vi "Teleop.vi"(10 "Match Info":T1={"Autonomous Elapsed Seconds"=0.0, "TeleOp Elapsed Seconds"=0.0, "Disabled Elapsed Seconds"=0.0, "Visited Autonomous"=FALSE, "Visited TeleOp"=FALSE, "Visited Disabled"=FALSE, "Autonomous Settings"={"Autonomous Style"=enum."Independent", "VI Refnum"=refnum}}, 11 "Call Context":T2) -> ()   [LabVIEW 2016]
doc: "This VI is called for each TeleOp packet received from the DS where the robot is not disabled. It is often used to read from the joysticks and update I/O or to update setpoints for timed control loops. It should complete and return within 20 milliseconds or it may miss DS packets."
uses:
  <vilib>/Rock Robotics/WPI/DriverStation/WPI_DriverStationDerivedRobotMode.ctl
  <vilib>/Rock Robotics/WPI/DriverStation/WPI_DriverStationMatch Info.ctl
  <vilib>/Rock Robotics/WPI/Relay/WPI_RelayValue.ctl
  <vilib>/Rock Robotics/WPI/Utilities/WPI_GetSetVariantRefNum.vi
  <vilib>/Rock Robotics/Network Tables/NT Write Boolean Array.vi
  <vilib>/Rock Robotics/Network Tables/NT Write Numeric Array.vi
  <vilib>/Rock Robotics/Network Tables/NT Read Boolean.vi
  <vilib>/Rock Robotics/Network Tables/NT Read Number.vi
  Robot Global Data.vi
panel:
  out "size y (1-200)":dbl
  out "center y (0-119)":dbl
  out "x+1":i32
  out "Sample Slider 0":dbl(slide) scale=0.0..5.0
  out "Sample Boolean 1":bool
  out "Sample Boolean 0":bool
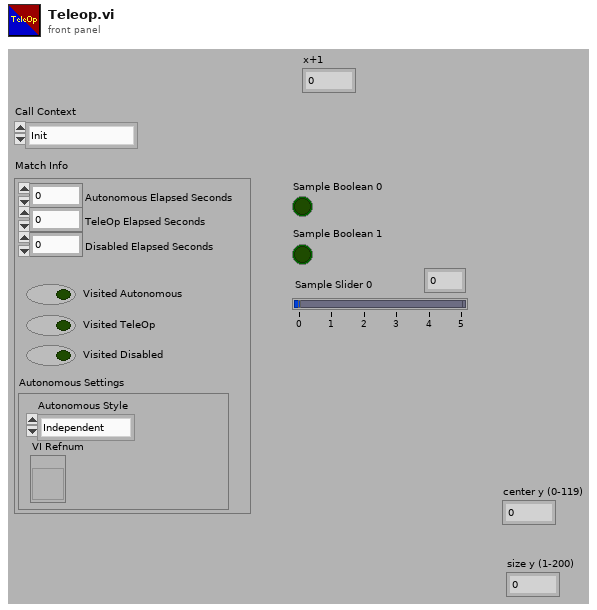
[diagram p1: front panel]
types:
  T1 = typedef "WPI_DriverStationMatch Info.ctl" = cluster{"Autonomous Elapsed Seconds":dbl, "TeleOp Elapsed Seconds":dbl, "Disabled Elapsed Seconds":dbl, "Visited Autonomous":bool, "Visited TeleOp":bool, "Visited Disabled":bool, "Autonomous Settings":cluster{"Autonomous Style":enum16{"Iterative", "Independent"}, "VI Refnum":refnum<vi>}}
  T2 = typedef "WPI_DriverStationDerivedRobotMode.ctl" = enum16{"Init", "Execute", "Stop"}
  T3 = typedef "WPI_RelayValue.ctl" = enum16{"Off", "On", "Forward", "Reverse"}
  T4 = typedef "WPI_JoystickDevRef.ctl" = cluster{"Device":T5}
  T5 = typedef "WPI_JoystickDeviceEnum.ctl" = enum16{"USB 0", "USB 1", "USB 2", "USB 3", "USB 4", "USB 5"}
  T6 = cluster{"Axes[0]":dbl, "Axes[1]":dbl, "Axes[2]":dbl, "Axes[3]":dbl, "Axes[4]":dbl, "Axes[5]":dbl, "Axes[6]":dbl, "Axes[7]":dbl, "Axes[8]":dbl}
  T7 = cluster{"Buttons[0]":bool, "Buttons[1]":bool, "Buttons[2]":bool, "Buttons[3]":bool, "Buttons[4]":bool, "Buttons[5]":bool, "Buttons[6]":bool, "Buttons[7]":bool, "Buttons[8]":bool}
  T8 = typedef "WPI_MotorControlDeviceRef.ctl" = cluster{"DeviceStatus":errorcluster, "Type":T9, "PWM":cluster{"PWM Channel":T10, "DeadBand":T11}, "CAN":cluster{"Device Number":u8, "SetOutput VI Ref":variant, "GetOutput VI Ref":variant, "Enable VI Ref":variant, "Disable VI Ref":variant, "Data":variant}, "Invert":bool}
  T9 = typedef "WPI_MotorControlType.ctl" = enum16{"PWM", "CAN"}
  T10 = typedef "FPGA_DIOPWMChannel.ctl" = enum8{"PWM 0", "PWM 1", "PWM 2", "PWM 3", "PWM 4", "PWM 5", "PWM 6", "PWM 7", "PWM 8", "PWM 9", "PWM MXP 0", "PWM MXP 1", "PWM MXP 2", "PWM MXP 3", "PWM MXP 4", "PWM MXP 5", "PWM MXP 6", "PWM MXP 7", "PWM MXP 8", "PWM MXP 9", "Invalid"}
  T11 = typedef "WPI_PWMDeadband.ctl" = cluster{"Name":string, "maxPositivePwm":i32, "minPositivePwm":i32, "centerPwm":i32, "maxNegativePwm":i32, "minNegativePwm":i32, "angularRange":u16}
  T12 = typedef "WPI_RelayDevRef.ctl" = cluster{"DevStatus":errorcluster, "Relay Channel":T13, "Relay Direction":T14}
  T13 = typedef "FPGA_DIORelayChannel.ctl" = enum8{"Relay 0", "Relay 1", "Relay 2", "Relay 3", "Invalid"}
  T14 = typedef "WPI_RelayDirection.ctl" = enum16{"Both directions", "Forward only", "Reverse only"}
  T15 = typedef "WPI_RobotDriveDevRef.ctl" = cluster{"DevStatus":errorcluster, "Motors[]":T8[], "Square Inputs":bool, "Max Output":dbl}
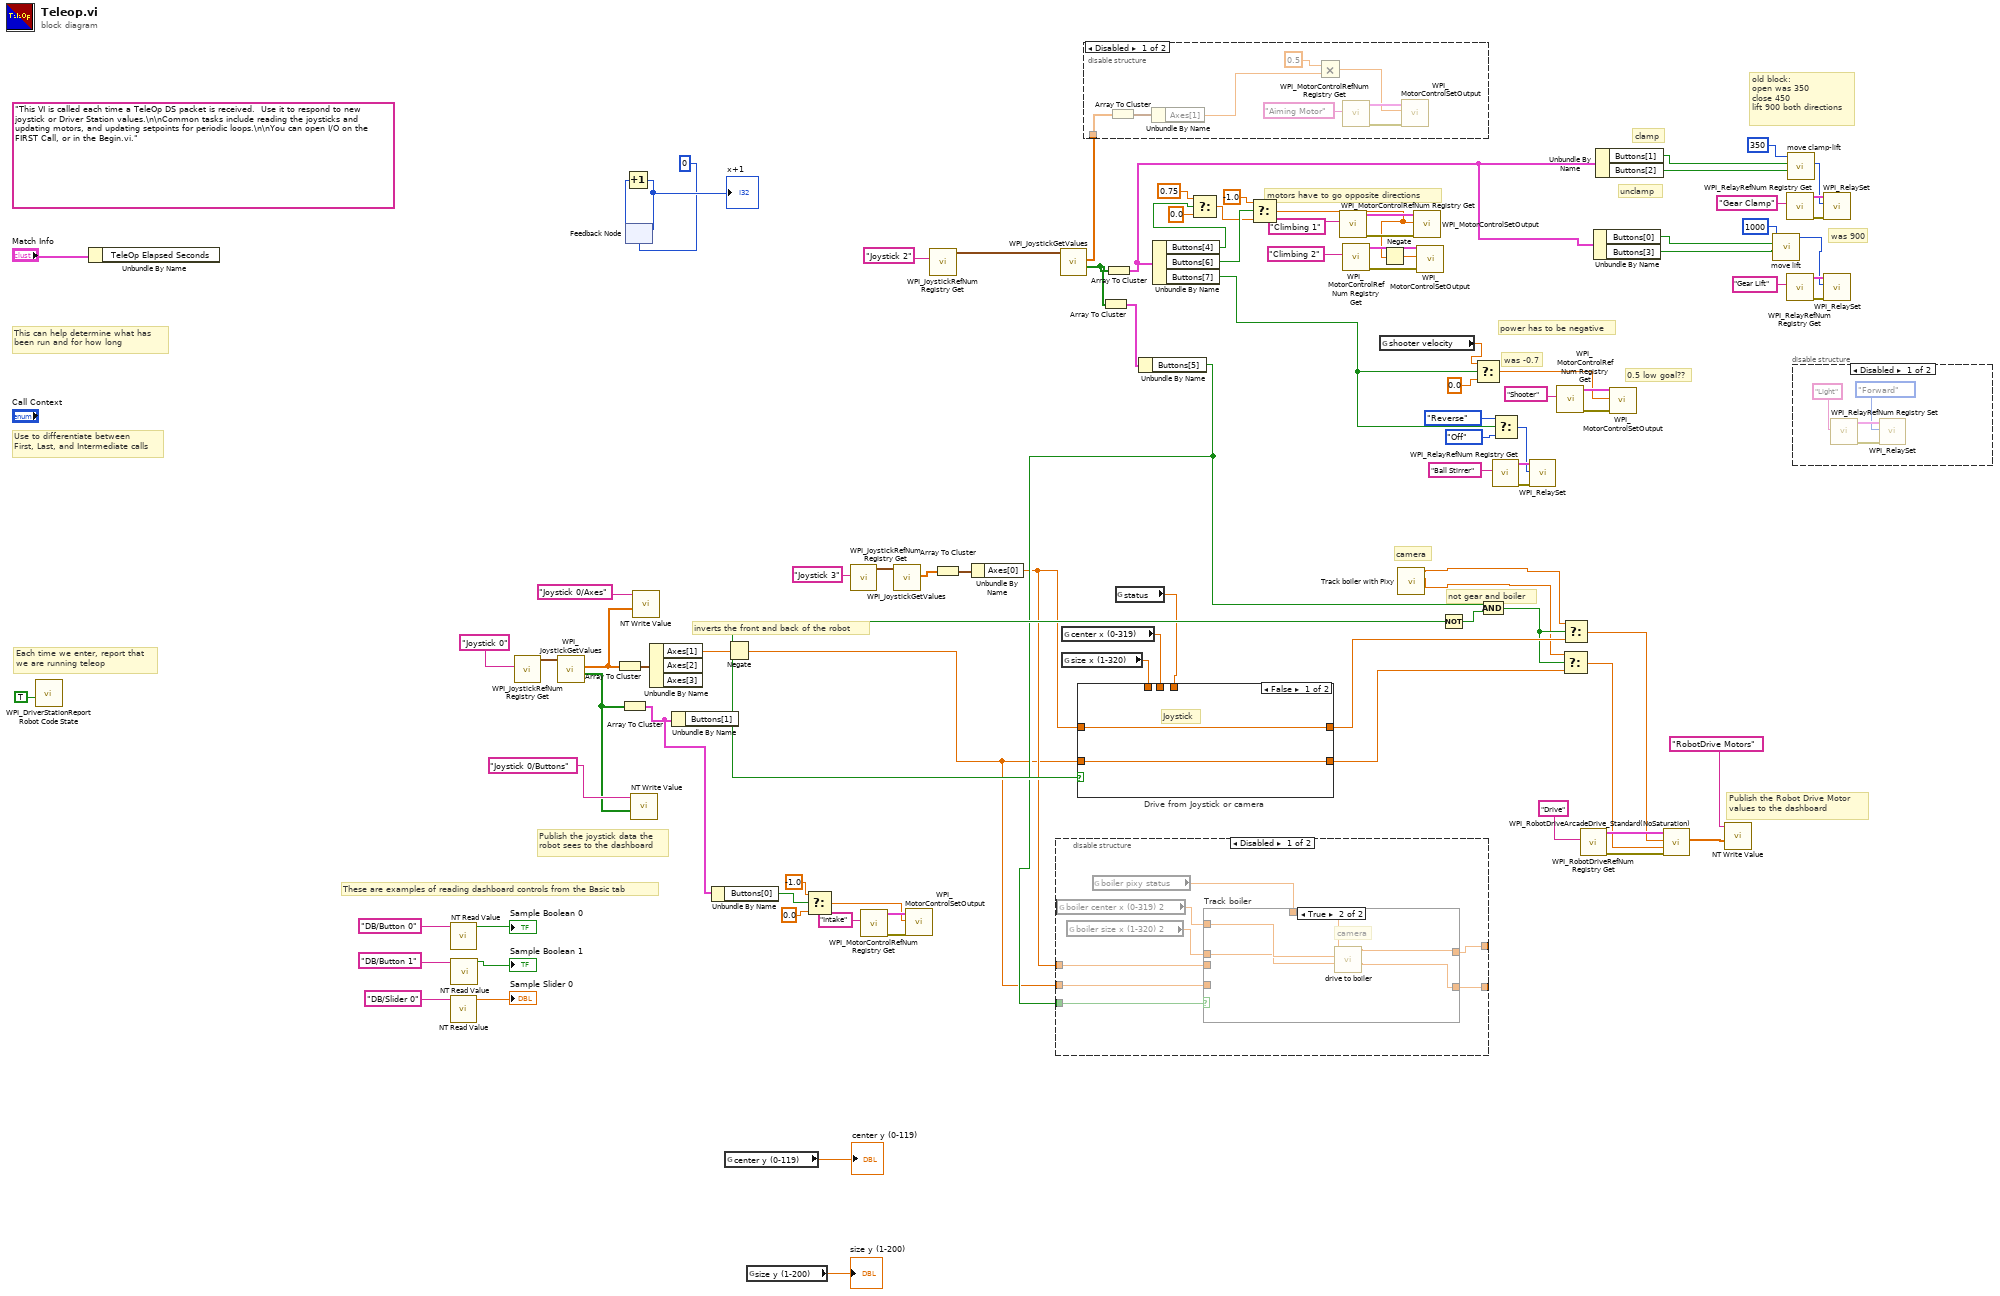
[diagram p0: block diagram]
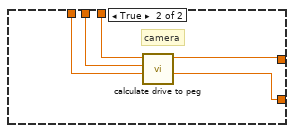
[diagram p6: hidden frame]
diagram:
  (unwired) "This VI is called each time a TeleOp DS packet is received.  Use it to respond to new joystick or Driver Station values.\n\nCommon tasks include reading the joysticks and updating motors, and updating setpoints for periodic loops.\n\nYou can open I/O on the FIRST Call, or in the Begin.vi."
  # "camera"
  # "not gear and boiler"
  # "was 900"
  # "old block:\nopen was 350\nclose 450\nlift 900 both directions"
  # "inverts the front and back of the robot"
  # "unclamp"
  # "clamp"
  # "was -0.7"
  # "0.5 low goal??"
  # "power has to be negative"
  # "motors have to go opposite directions"
  # "These are examples of reading dashboard controls from the Basic tab"
  # "Publish the Robot Drive Motor\nvalues to the dashboard"
  # "Publish the joystick data the\nrobot sees to the dashboard"
  # "Each time we enter, report that\nwe are running teleop"
  # "Use to differentiate between\nFirst, Last, and Intermediate calls"
  # "This can help determine what has\nbeen run and for how long"
  n1 = call <vilib>:"WPI_DriverStationReport Robot Code State.vi"("TeleOp"=TRUE ("Autonomous")) -> ()  [unwired: 10 in, 1 out]
  n2 = Unbundle By Name("Match Info") -> ()  [unwired: 1 out]
  n3 = call-poly <vilib>:"NT Read Value.vi"("Name"="DB/Button 0" ("refnum name")) -> ("Boolean"=→"Sample Boolean 0":bool)  [unwired: 9 in, 1 out]
  n4 = call-poly <vilib>:"NT Read Value.vi"("Name"="DB/Slider 0" ("refnum name")) -> ("Numeric"=→"Sample Slider 0":dbl)  [unwired: 9 in, 1 out]
  n5 = call-poly <vilib>:"NT Read Value.vi"("Name"="DB/Button 1" ("refnum name")) -> ("Boolean"=→"Sample Boolean 1":bool)  [unwired: 9 in, 1 out]
  n6 = call <vilib>:"WPI_JoystickRefNum Registry Get.vi"("refnum name"="Joystick 0") -> ("JoystickDevRef"=w96:T4)  [unwired: 1 in, 9 out]
  n7 = call <vilib>:"WPI_JoystickGetValues.vi"("JoystickDevRef"=w96) -> ("Buttons"=w84:bool[], "Axes"=w85:dbl[])  [unwired: 6 in, 3 out]
  n8 = Array To Cluster(array=w85) -> (cluster=w86:T6)
  n9 = Array To Cluster(array=w84) -> (cluster=w35:T7)
  n10 = feedback #1(0) -> (w75:i32)
  n11 = Increment(x=w75) -> (x+1=w76:i32)
  "x+1" <- w76
  n12 = feedback-in #1(w76) -> ()
  n13 = call-poly <vilib>:"NT Write Value.vi"("Boolean Array"=w84, "Name"="Joystick 0/Buttons") -> ()  [unwired: 9 in, 1 out]
  n14 = call-poly <vilib>:"NT Write Value.vi"("Numeric Array"=w85, "Name"="Joystick 0/Axes") -> ()  [unwired: 9 in, 1 out]
  n15 = Unbundle By Name(w86) -> ("Axes[1]"=w73:dbl)  [unwired: 2 out]
  n16 = Unbundle By Name(w35) -> ("Buttons[1]"=w20:bool)
  n17 = Unbundle By Name(w35) -> ("Buttons[0]"=w33:bool)
  n18 = global read "Robot Global Data.vi" "center y (0-119)"() -> (→"center y (0-119)":dbl)
  n19 = Negate(x=w73) -> (-x=w13:dbl)
  n20 = global read "Robot Global Data.vi" "size y (1-200)"() -> (→"size y (1-200)":dbl)
  n21 = Select(t=-1.0, s=w33, f=0.0) -> (s? t:f=w78:dbl)
  n22 = call <vilib>:"WPI_JoystickRefNum Registry Get.vi"("refnum name"="Joystick 3") -> ("JoystickDevRef"=w45:T4)  [unwired: 1 in, 9 out]
  n23 = call <vilib>:"WPI_MotorControlRefNum Registry Get.vi"("refnum name"="Intake") -> ("error out"=w81:errorcluster, "MotorControlDevRef"=w80:T8)  [unwired: 9 in]
  n24 = call <vilib>:"WPI_JoystickGetValues.vi"("JoystickDevRef"=w45) -> ("Axes"=w44:dbl[])  [unwired: 6 in, 4 out]
  n25 = call <vilib>:"WPI_MotorControlSetOutput.vi"("error in (no error)"=w81, "Output"=w78, "MotorControlDevRef"=w80) -> ()  [unwired: 6 in, 3 out]
  n26 = call <vilib>:"WPI_JoystickRefNum Registry Get.vi"("refnum name"="Joystick 2") -> ("JoystickDevRef"=w68:T4)  [unwired: 1 in, 9 out]
  n27 = Array To Cluster(array=w44) -> (cluster=w43:T6)
  n28 = Unbundle By Name(w43) -> ("Axes[0]"=w14:dbl)
  n29 = call <vilib>:"WPI_JoystickGetValues.vi"("JoystickDevRef"=w68) -> ("Buttons"=w19:bool[], "Axes"=w60:dbl[])  [unwired: 6 in, 3 out]
  n30 = global read "Robot Global Data.vi" "center x (0-319)"() -> (w11:dbl)
  n31 = global read "Robot Global Data.vi" "size x (1-320)"() -> (w10:dbl)
  n32 = disable-structure shown="Disabled" {
    disable-tunnel: w60 -> [w108 _]
    frame Disabled {
      n33 = Array To Cluster(array=w108) -> (cluster=w107:T6)
      n34 = Unbundle By Name(w107) -> ("Axes[1]"=w101:dbl)
      n35 = Multiply(x=0.5 ("y"), y=w101) -> (x*y=w103:dbl)
      n36 = call <vilib>:"WPI_MotorControlRefNum Registry Get.vi"("refnum name"="Aiming Motor") -> ("error out"=w104:errorcluster, "MotorControlDevRef"=w105:T8)  [unwired: 9 in]
      n37 = call <vilib>:"WPI_MotorControlSetOutput.vi"("error in (no error)"=w104, "Output"=w103, "MotorControlDevRef"=w105) -> ()  [unwired: 6 in, 3 out]
    }
    frame Enabled {
    }
  }
  n38 = Array To Cluster(array=w19) -> (cluster=w16:T7)
  n39 = Array To Cluster(array=w19) -> (cluster=w18:T7)
  n40 = global read "Robot Global Data.vi" "status"() -> (w12:dbl)
  n41 = case "Drive from Joystick or camera" shown="False" w20 {
    tunnel: w14 -> [w110 _]
    tunnel: [w110 w115] -> w9
    tunnel: w13 -> [w109 _]
    tunnel: [w109 w114] -> w8
    tunnel: w12 -> [_ w113]
    tunnel: w11 -> [_ w112]
    tunnel: w10 -> [_ w111]
    frame False {
      # "Joystick"
    }
    frame True {
      # "camera"
      n42 = call "calculate drive to peg.vi"("status"=w113, "center x (0-319)"=w112, "size x (1-320)"=w111) -> ("x"=w115:dbl, "y"=w114:dbl)  [unwired: 6 in]
    }
  }
  n43 = Unbundle By Name(w16) -> ("Buttons[5]"=w15:bool)
  n44 = disable-structure shown="Disabled" {
    disable-tunnel: w15 -> [w120 _]
    disable-tunnel: [w119 _] -> _
    disable-tunnel: [w118 _] -> _
    disable-tunnel: w14 -> [w117 _]
    disable-tunnel: w13 -> [w116 _]
    frame Disabled {
      n45 = global read "Robot Global Data.vi" "boiler center x (0-319) 2"() -> (w122:dbl)
      n46 = global read "Robot Global Data.vi" "boiler size x (1-320) 2"() -> (w121:dbl)
      n47 = global read "Robot Global Data.vi" "boiler pixy status"() -> (w123:dbl)
      n48 = case "Track boiler" shown="True" w120 {
        tunnel: [w125 w130] -> w119
        tunnel: [w124 w129] -> w118
        tunnel: w123 -> [_ w128]
        tunnel: w122 -> [_ w127]
        tunnel: w121 -> [_ w126]
        tunnel: w117 -> [w125 _]
        tunnel: w116 -> [w124 _]
        frame False {
          # "Joystick"
        }
        frame True {
          # "camera"
          n49 = call "drive to boiler.vi"(9:w126, 10:w127, 11:w128) -> ("y output"=w129:dbl, "x output"=w130:dbl)  [unwired: 7 in]
        }
      }
    }
    frame Enabled {
    }
  }
  n50 = Unbundle By Name(w18) -> ("Buttons[4]"=w27:bool, "Buttons[6]"=w41:bool, "Buttons[7]"=w17:bool)
  n51 = Select(t=0.75, s=w27, f=0.0) -> (s? t:f=w25:dbl)
  n52 = Select(t=-1.0, s=w41, f=w25) -> (s? t:f=w36:dbl)
  n53 = call <vilib>:"WPI_MotorControlRefNum Registry Get.vi"("refnum name"="Climbing 1") -> ("error out"=w66:errorcluster, "MotorControlDevRef"=w65:T8)  [unwired: 9 in]
  n54 = call <vilib>:"WPI_MotorControlRefNum Registry Get.vi"("refnum name"="Climbing 2") -> ("error out"=w63:errorcluster, "MotorControlDevRef"=w64:T8)  [unwired: 9 in]
  n55 = global read "Robot Global Data.vi" "shooter velocity"() -> (w1:dbl)
  n56 = Negate(x=w36) -> (-x=w37:dbl)
  n57 = call "Track boiler with Pixy.vi"() -> ("y output"=w4:dbl, "x output"=w5:dbl)  [unwired: 7 in, 2 out]
  n58 = call <vilib>:"WPI_MotorControlSetOutput.vi"("error in (no error)"=w66, "Output"=w36, "MotorControlDevRef"=w65) -> ()  [unwired: 6 in, 3 out]
  n59 = call <vilib>:"WPI_MotorControlSetOutput.vi"("error in (no error)"=w63, "Output"=w37, "MotorControlDevRef"=w64) -> ()  [unwired: 6 in, 3 out]
  n60 = Not(x=w20) -> (.not. x?=w6:bool)
  n61 = Select(t=w1, s=w17, f=0.0) -> (s? t:f=w56:dbl)
  n62 = And(x=w15, y=w6) -> (x .and. y?=w7:bool)
  n63 = call <vilib>:"WPI_RelayRefNum Registry Get.vi"("refnum name"="Ball Stirrer") -> ("error out"=w54:errorcluster, "RelayDevRef"=w53:T12)  [unwired: 9 in]
  n64 = Select(t=WPI_RelayValue."Reverse" ("RelayValue"), s=w17, f=WPI_RelayValue."Off" ("RelayValue")) -> (s? t:f=w52:T3)
  n65 = call <vilib>:"WPI_RelaySet.vi"("error in (no error)"=w54, "RelayValue"=w52, "RelayDevRef"=w53) -> ()  [unwired: 7 in, 2 out]
  n66 = call <vilib>:"WPI_MotorControlRefNum Registry Get.vi"("refnum name"="Shooter") -> ("error out"=w59:errorcluster, "MotorControlDevRef"=w58:T8)  [unwired: 9 in]
  n67 = Select(t=w4, s=w7, f=w8) -> (s? t:f=w2:dbl)
  n68 = Select(t=w5, s=w7, f=w9) -> (s? t:f=w3:dbl)
  n69 = call <vilib>:"WPI_RobotDriveRefNum Registry Get.vi"("refnum name"="Drive") -> ("error out"=w34:errorcluster, "RobotDriveDevRef"=w98:T15)  [unwired: 1 in, 8 out]
  n70 = Unbundle By Name(w18) -> ("Buttons[0]"=w23:bool, "Buttons[3]"=w22:bool)
  n71 = Unbundle By Name(w18) -> ("Buttons[1]"=w31:bool, "Buttons[2]"=w30:bool)
  n72 = call <vilib>:"WPI_MotorControlSetOutput.vi"("error in (no error)"=w59, "Output"=w56, "MotorControlDevRef"=w58) -> ()  [unwired: 6 in, 3 out]
  n73 = call <vilib>:"WPI_RobotDriveArcadeDrive_Standard(NoSaturation).vi"("error in (no error)"=w34, "Y axis value"=w2, "X axis value"=w3, "RobotDriveDevRef"=w98) -> ("Motor Values"=w70:dbl[])  [unwired: 7 out]
  n74 = call-poly <vilib>:"NT Write Value.vi"("Numeric Array"=w70, "Name"="RobotDrive Motors") -> ()  [unwired: 9 in, 1 out]
  n75 = call "move lift.vi"("button 3"=w22, "button 0"=w23, "time"=u32 1000 ("forward time")) -> ("output"=w24:T3)  [unwired: 8 in]
  n76 = call <vilib>:"WPI_RelayRefNum Registry Get.vi"("refnum name"="Gear Clamp") -> ("error out"=w48:errorcluster, "RelayDevRef"=w47:T12)  [unwired: 9 in]
  n77 = call <vilib>:"WPI_RelayRefNum Registry Get.vi"("refnum name"="Gear Lift") -> ("error out"=w38:errorcluster, "RelayDevRef"=w39:T12)  [unwired: 9 in]
  n78 = call "move clamp-lift.vi"("button 2"=w30, "button 1"=w31, "time"=u32 350 ("forward time")) -> ("output"=w29:T3)  [unwired: 8 in]
  n79 = disable-structure shown="Disabled" {
    frame Disabled {
      n80 = call <vilib>:"WPI_RelayRefNum Registry Set.vi"("refnum name"="Light") -> ("error out"=w133:errorcluster, "RelayDevRef"=w132:T12)  [unwired: 9 in]
      n81 = call <vilib>:"WPI_RelaySet.vi"("error in (no error)"=w133, "RelayValue"=WPI_RelayValue."Forward", "RelayDevRef"=w132) -> ()  [unwired: 7 in, 2 out]
    }
    frame Enabled {
    }
  }
  n82 = call <vilib>:"WPI_RelaySet.vi"("error in (no error)"=w48, "RelayValue"=w29, "RelayDevRef"=w47) -> ()  [unwired: 7 in, 2 out]
  n83 = call <vilib>:"WPI_RelaySet.vi"("error in (no error)"=w38, "RelayValue"=w24, "RelayDevRef"=w39) -> ()  [unwired: 7 in, 2 out]
